vi "Configure Step Connect Mode.vi"(0 "VISA resource name":refnum<visa-resource-name>, 5 "Enable Step Connection (F:Disable)":bool, 11 "error in (no error)":errorcluster) -> (4 "VISA resource name out":refnum<visa-resource-name>, 15 "error out":errorcluster)   [LabVIEW 2016, in "APT 300XAC Series.lvlib"]
doc: "Sets the <B>Step Connect mode</B> of the active step in the current Memory location (Use \"Configure Memory.vi\" to select the desired memory)\n\n<B>Range</B> : [Disable : Stop Sequence ,Enable : Go to next step]\n\nThe step connect parameter setting configures whether one step will be linked or connected to another step. For example in order to links step one to step two the connect must be Enabled. Steps can only be connected in sequential order."
uses:
  APT 300XAC Series.lvlib
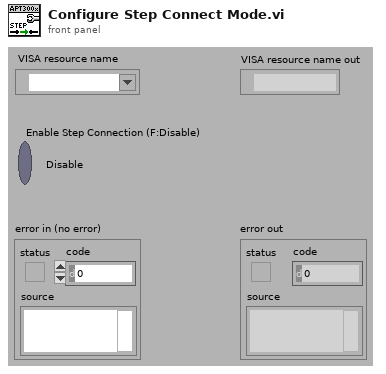
[diagram p1: front panel]
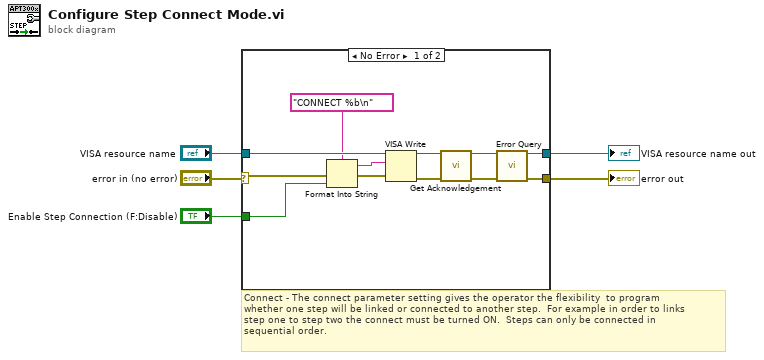
[diagram p0: block diagram]
diagram:
  # "Connect - The connect parameter setting gives the operator the flexibility  to program \nwhether one step will be linked or connected to another step.  For example in order to links \nstep one to step two the connect must be turned ON.  Steps can only be connected in \nsequential order."
  n1 = case shown="No Error" "error in (no error)" {
    selector: "error in (no error)" -> [w12 w19]
    tunnel: "VISA resource name" -> [w17 w18]
    tunnel: [w14 w18] -> w4
    tunnel: [w13 w19] -> w3
    tunnel: "Enable Step Connection (F:Disable)" -> [w10 _]
    frame No Error {
      n2 = Format Into String(format string="CONNECT %b\n" ("Command"), error in=w12, w10) -> (resulting string=w16:string, error out=w11:errorcluster)  [unwired: 1 in]
      n3 = VISA Write(VISA resource name=w17, write buffer=w16, error in (no error)=w11) -> (VISA resource name out=w7:refnum<visa-resource-name>, error out=w6:errorcluster)  [unwired: 1 out]
      n4 = call "Get Acknowledgement.vi"("VISA resource name"=w7, "error in (no error)"=w6) -> ("VISA resource name out"=w8:refnum<visa-resource-name>, "error out"=w9:errorcluster)  [unwired: 12 in]
      n5 = call "Error Query.vi"("VISA resource name"=w8, "error in (no error)"=w9) -> ("VISA resource name out"=w14:refnum<visa-resource-name>, "error out"=w13:errorcluster)  [unwired: 10 in, 2 out]
    }
    frame Error {
    }
  }
  "error out" <- w3
  "VISA resource name out" <- w4
